vi "sv_Fractional-octave Analysis (N Ch).vi"(0 "Scaled signal(s)":waveform(dbl)[](array[waveform]), 1 "1/n octave settings":T7={"standard"=enum."ANSI S1.11", "bandwidth"=enum."1/3 octave"}, 5 "band number":cluster{"low band":i32, "high band":i32}, 7 "restart averaging (F)":bool, 9 "reset filter (F)":bool, 11 "error in (no error)":errorcluster, 12 "averaging type":T8(ring), 13 "exp avg settings":T5={" mode"=enum."Fast", "time constant [ms]"=125.0} {"time constant [ms]" format="%.2f"}, 14 "equal confidence level [dB]":dbl=125.0 format="%.2f") -> (3 "settled?":bool, 4 "Octave measurements":T6(array[cluster]) {"band power [EU^2 rms]" format="%.2f"; "dup nominal frequencies [Hz" format="%.2f"}, 6 "# samples to settle":u64, 10 "octave info":T1[](array[typedef]) {"engineering units" items=["custom..."=0, "V"=1, "A"=21, "C"=30, "pC"=31, "s"=32, "-"=29, "Pa"=2, "N"=20, "g"=3, "m/s^2"=4, "m/s"=5, "m"=6, "mm/s"=12, "mm"=13, "micron/s"=14, "micron"=15, "in/s^2"=7, "in/s"=8, "in"=9, "mil/s"=10, "mil"=11, "rad/s^2"=16, "rad/s"=17, "rad"=18, "deg/s^2"=26, "deg/s"=27, "deg"=28, "RPM"=22, "cycle/s^2"=23, "Hz"=24, "cycle"=25, "strain"=19]; "dB reference" format="%.2e"; "weighting filter" items=["Linear", "A-weighting", "B-weighting", "C-weighting", "ITU-R 468-4", "Dolby", "CCITT", "C-message", "Wb", "Wc", "Wd", "We", "Wf", "Wh", "Wj", "Wk", "Wm", "AES17 20 kHz lowpass", "AES17 40 kHz lowpass", "AES17 20 kHz highpass", "AES17 40 kHz highpass"]}, 15 "error out":errorcluster)   [LabVIEW 2017, in "SoundVib_Octave.lvlib"]
doc: "Performs a fractional-octave analysis on the input signal.\nThe fractional-octave filters are designed in accordance with one of the following standards:\n ANSI S1.11-1986, Order 3, Type 1-D, optional range;\n Fractional-octave-band filters, class 1, IEC 1260:1995.\nFor both standards, the sampling frequency must be at least 3 times the highest midband frequency for octave analysis and at least 2.5 times the highest midband frequency for 1/3, 1/6, 1/12, or 1/24 octave analysis. Available bandwidths are 1/1, 1/3, 1/6, 1/12, and 1/24 octave.\nThe frequency range is based on the low and high bands specified in the band number cluster. A value of 0 corresponds to the reference frequency of the audio-frequency \nrange 1 kHz. Each successive value corresponds to the next fractional-octave band. Positive values cover the range above 1 kHz, and negative values cover the range below 1 kHz.\nAvailable averaging types are Linear, Exponential (default), Equal confidence, and Peak. Based on the selected averaging type, this VI uses the additional settings in averaging parameters.\nThis VI returns the power in each fractional-octave band.\nTo ensure a continuous filtering operation call this VI the first time with filter init/cont set to FALSE and then call it with filter init/cont set to TRUE."
uses:
  <vilib>/addons/Sound and Vibration/svt_Octave/SoundVib_Octave.lvlib
  <vilib>/addons/_NISVFA/_Shared subVIs/Controls/svc_Octave Standard.ctl
  <vilib>/addons/_NISVFA/_Shared subVIs/Controls/svc_Octave Info.ctl
  <vilib>/addons/_NISVFA/_Shared subVIs/Controls/svc_Weighting Filter Text Ring.ctl
  <vilib>/addons/_NISVFA/_Shared subVIs/Controls/svc_Engineering Units Text Ring.ctl
  <vilib>/addons/Sound and Vibration/svt_Octave_2014 standard/SoundVib_Octave_2014 standard.lvlib
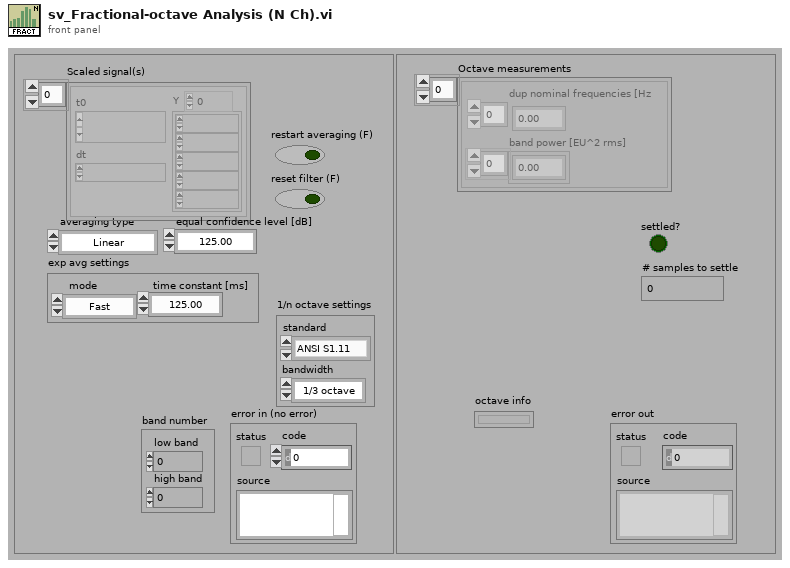
[diagram p1: front panel]
types:
  T1 = typedef "svc_Octave Info.ctl" = cluster{"standard":T2, "bandwidth":enum16{"1 octave", "1/3 octave", "1/6 octave", "1/12 octave", "1/24 octave"}, "low band":i32, "high band":i32, "weighting filter":T3, "dB reference":dbl, "dB On":bool, "unit label":string, "channel name":string, "description":string, "engineering units":T4, "custom label":string, "spectrum type":enum16{"power", "magnitude"}, "spectral density":bool, "filters settled":bool}
  T2 = typedef "svc_Octave Standard.ctl" = enum16{"ANSI S1.11", "IEC 61260"}
  T3 = typedef "svc_Weighting Filter Text Ring.ctl" = u16
  T4 = typedef "svc_Engineering Units Text Ring.ctl" = u16
  T5 = cluster{" mode":enum16{"Slow", "Fast", "Impulse", "Custom"}, "time constant [ms]":dbl}
  T6 = cluster{"dup nominal frequencies [Hz":dbl[], "band power [EU^2 rms]":dbl[]}[]
  T7 = cluster{"standard":T2, "bandwidth":enum16{"1 octave", "1/3 octave", "1/6 octave", "1/12 octave", "1/24 octave"}}
  T8 = enum16{"Linear", "Exponential", "Equal confidence", "Peak"}
  T9 = enum16{"1 octave", "1/3 octave", "1/6 octave", "1/12 octave", "1/24 octave", "1/48 octave", "1/96 octave"}
  T10 = cluster{"# special filters":i32, "special filter coefficients":cluster{"filter structure":enum32{"IIR 2nd Order", "IIR 4th Order"}, "Reverse Coefficients":dbl[], "Forward Coefficients":dbl[]}[], "# filters per octave":cluster{"# filters":i32, "starting at":i32}[], "standard filter coefficients":cluster{"filter structure":enum32{"IIR 2nd Order", "IIR 4th Order"}, "Reverse Coefficients":dbl[], "Forward Coefficients":dbl[]}[], "# decimation steps":i32, "lowpass filter coefficients":cluster{"filter structure":enum32{"IIR 2nd Order", "IIR 4th Order"}, "Reverse Coefficients":dbl[], "Forward Coefficients":dbl[]}, "# samples to settle":u64, "special filter bandwidth":dbl[], "standard filter bandwidth":dbl[]}
  T11 = cluster{"octave filter":cluster{"Octave filter":dbl[]}[], "decimation":i32[], "lowpass filter":dbl[][], "exponential averaging":cluster{"exponential averaging":dbl, "peak detector":dbl}[], "linear averaging":cluster{"squared sum":dbl, "size":dbl}[], "result":dbl[], "# samples since init":u64}
  T12 = cluster{"octave filter":cluster{"Octave filter":dbl[]}[], "decimation":i32[], "lowpass filter":dbl[][], "exponential averaging":cluster{"exponential averaging":dbl, "peak detector":dbl}[], "linear averaging":cluster{"squared sum":dbl, "size":dbl}[], "result":dbl[], "# samples since init":u64}[]
  T13 = enum16{"1 octave", "1/3 octave", "1/6 octave", "1/12 octave", "1/24 octave"}
  T14 = cluster{"dup nominal frequencies [Hz":dbl[], "band power [EU^2 rms]":dbl[]}
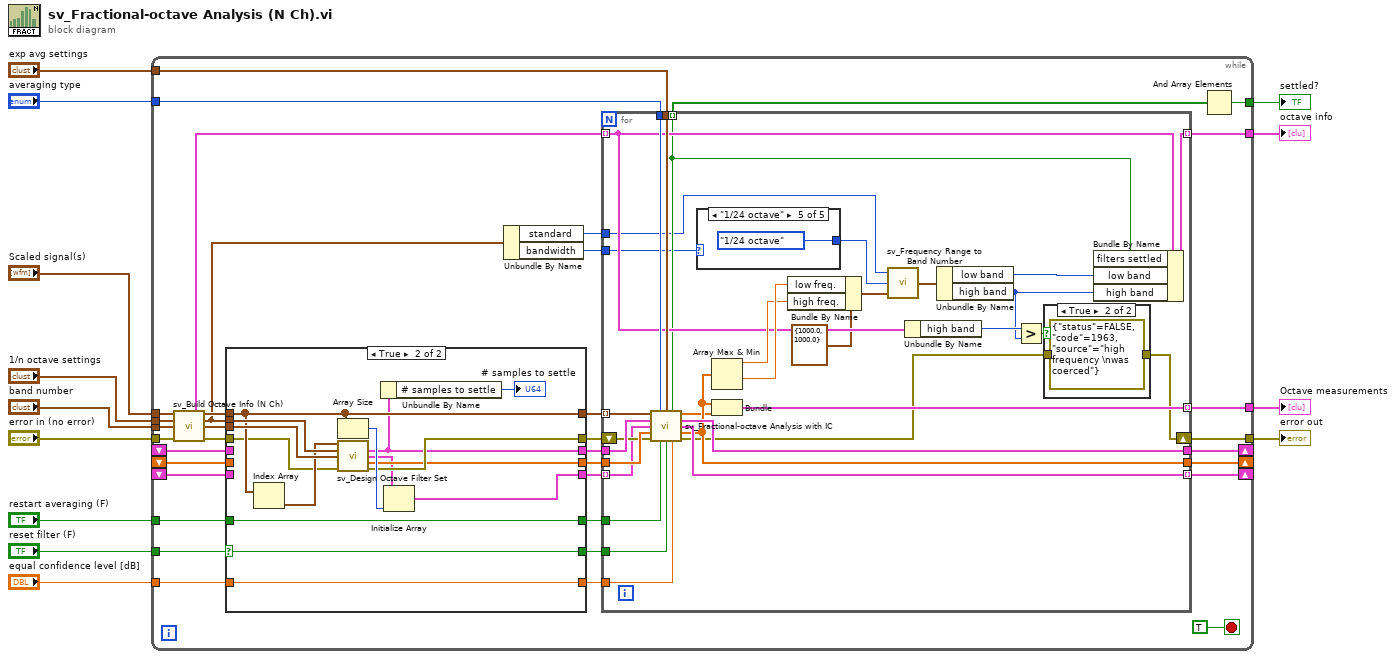
[diagram p0: block diagram]
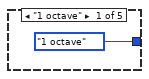
[diagram p2: hidden frame]
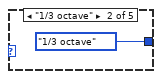
[diagram p3: hidden frame]
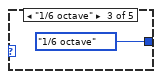
[diagram p4: hidden frame]
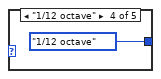
[diagram p5: hidden frame]
diagram:
  n1 = while {
    tunnel: [w22] -> w1
    tunnel: [w23] -> w2
    tunnel: [w17] -> w3
    tunnel: "error in (no error)" -> [w28]
    tunnel: "band number" -> [w30]
    tunnel: "1/n octave settings" -> [w31]
    tunnel: "equal confidence level [dB]" -> [w26]
    tunnel: "exp avg settings" -> [w34]
    tunnel: "averaging type" -> [w38]
    tunnel: [w39] -> w10
    shift-left: _ -> [w40]
    shift-right: [w41] -> _
    shift-left: _ -> [w42]
    shift-right: [w43] -> _
    shift-left: _ -> [w46]
    shift-right: [w20] -> _
    tunnel: "restart averaging (F)" -> [w36]
    tunnel: "Scaled signal(s)" -> [w32]
    tunnel: "reset filter (F)" -> [w48]
    stop <- TRUE stop-if-true
    n2 = call <vilib>:"sv_Build Octave Info (N Ch).vi"("scaled signals"=w32, "1/n octave settings"=w31, "band number"=w30, "error in (no error)"=w28) -> ("octave info"=w19:T1[], "scaled signals"=w33:waveform(dbl)[], "dup 1/n octave settings"=w16:T7, "dup band number"=w29:cluster{"low band":i32, "high band":i32}, "error out"=w27:errorcluster)  [unwired: 7 in]
    n3 = case shown="True" w48 {
      selector: w48 -> [w96 w111]
      tunnel: [w96 w111] -> w37
      tunnel: w33 -> [w95 w102]
      tunnel: [w93 w99] -> w44
      tunnel: [w95 w102] -> w47
      tunnel: [w90 w106] -> w24
      tunnel: [w92 w105] -> w45
      tunnel: w16 -> [_ w103]
      tunnel: w29 -> [_ w104]
      tunnel: [w94 w108] -> w21
      tunnel: w46 -> [w94 _]
      tunnel: w42 -> [w93 _]
      tunnel: w40 -> [w92 _]
      tunnel: [w91 w109] -> w35
      tunnel: w36 -> [w91 w109]
      tunnel: w27 -> [w90 w97]
      tunnel: w26 -> [w89 w107]
      tunnel: [w89 w107] -> w25
      frame False {
        # "Filter bank coefficients \nonly computed on reset"
      }
      frame True {
        n4 = Index Array(array=w102) -> (element=w101:waveform(dbl))  [unwired: 1 in]
        n5 = Array Size(array=w102) -> (size(s)=w110:i32)
        n6 = call <vilib>:"sv_Design Octave Filter Set.vi"("scaled signal [EU]"=w101, "1/n octave settings"=w103, "band number"=w104, "error in (no error)"=w97) -> ("filter bank parameters"=w99:T10, "initial filter state"=w100:T11, "nominal frequencies [Hz]"=w105:dbl[], "error out"=w106:errorcluster)  [unwired: 7 in, 1 out]
        n7 = Unbundle By Name(w99) -> ("# samples to settle"=→"# samples to settle":u64)
        n8 = Initialize Array(w100, w110) -> (w108:T12)
      }
    }
    n9 = Unbundle By Name(w16) -> ("standard"=w14:T2, "bandwidth"=w15:T13)
    n10 = for {
      tunnel: w47 -> [w72] mode=indexing
      tunnel: w45 -> [w81]
      tunnel: w44 -> [w80]
      tunnel: [w79] -> w43
      tunnel: [w63] -> w41
      tunnel: [w78] -> w39 mode=indexing
      tunnel: w38 -> [w77]
      tunnel: w37 -> [w76]
      tunnel: w35 -> [w75]
      tunnel: w34 -> [w74]
      tunnel: w25 -> [w73]
      shift-right: [w60] -> w23
      shift-left: w24 -> [w71]
      tunnel: [w54] -> w18 mode=indexing
      tunnel: w21 -> [w70] mode=indexing
      tunnel: [w69] -> w20 mode=indexing
      tunnel: w19 -> [w58] mode=indexing
      tunnel: [w61] -> w17 mode=indexing
      tunnel: w15 -> [w51]
      tunnel: w14 -> [w50]
      n11 = call <vilib>:"sv_Fractional-octave Analysis with IC.vi"("scaled signal [EU]"=w72, "averaging type"=w77, "exp avg settings"=w74, "filter bank parameters"=w80, "internal filter state IN"=w70, "nominal frequencies [Hz]"=w81, "error in (no error)"=w71, "restart averaging (F)"=w75, "reset filter"=w76, "equal confidence level [dB]"=w73) -> ("filter settled ?"=w54:bool, "band power [EU^2 rms]"=w62:dbl[], "dup filter bank parameters"=w79:T10, "internal filter state OUT"=w69:T11, "dup nominal frequencies [Hz"=w63:dbl[], "error out"=w59:errorcluster)
      n12 = case shown="\"1/24 octave\"" w51 {
        tunnel: [T9."1 octave" ("bandwidth") T9."1/3 octave" ("bandwidth") T9."1/6 octave" ("bandwidth") T9."1/12 octave" ("bandwidth") T9."1/24 octave" ("bandwidth")] -> w52
        frame "1 octave" {
        }
        frame "1/3 octave" {
        }
        frame "1/6 octave" {
        }
        frame "1/12 octave" {
        }
        frame "1/24 octave" {
        }
      }
      n13 = Array Max & Min(array=w63) -> (max value=w67:dbl, min value=w68:dbl)  [unwired: 2 out]
      n14 = Bundle("dup nominal frequencies [Hz"=w63, "band power [EU^2 rms]"=w62) -> (w78:T14)  [unwired: 1 in]
      n15 = Bundle By Name(cluster=cluster{"low freq.":dbl, "high freq.":dbl} {"low freq."=1000.0, "high freq."=1000.0} ("frequency range [Hz]"), "low freq."=w68, "high freq."=w67) -> (w66:cluster{"low freq.":dbl, "high freq.":dbl})
      n16 = call <vilib>:"sv_Frequency Range to Band Number.vi"("frequency range [Hz]"=w66, "bandwidth"=w52, "standard"=w50) -> ("band number"=w65:cluster{"low band":i32, "high band":i32})
      n17 = Unbundle By Name(w58) -> ("high band"=w57:i32)
      n18 = Unbundle By Name(w65) -> ("low band"=w64:i32, "high band"=w55:i32)
      n19 = Greater?(x=w57, y=w55) -> (0:w56:bool)
      n20 = case shown="True" w56 {
        tunnel: [w87 errorcluster {"status"=FALSE, "code"=1963, "source"="high frequency \nwas coerced"} ("error IO")] -> w60
        tunnel: w59 -> [w87 _]
        frame False {
        }
        frame True {
        }
      }
      n21 = Bundle By Name(cluster=w58, "filters settled"=w54, "low band"=w64, "high band"=w55) -> (w61:T1)
    }
    n22 = And Array Elements(Boolean array=w18) -> (logical AND=w22:bool)
  }
  "settled?" <- w1
  "error out" <- w2
  "Octave measurements" <- w10
  "octave info" <- w3
